vi "command change motor.vi"(8 "error in (no error)":errorcluster, 10 "the_command_change_motor":cluster{"Motor":u32}, 11 "id":i32) -> (0 "error out":errorcluster, 3 "function return":i32)   [LabVIEW 2012, in "libximc.lvlib"]
doc: "result_t XIMC_API command_change_motor (device_t id, const command_change_motor_t* the_command_change_motor);"
uses:
  libximc.lvlib
  libximc.dll
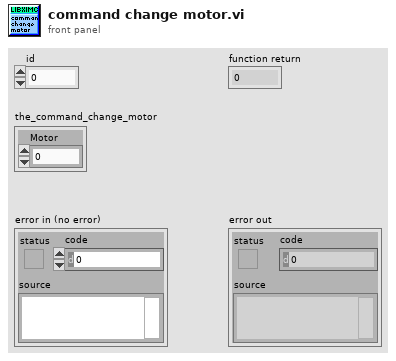
[diagram p1: front panel]
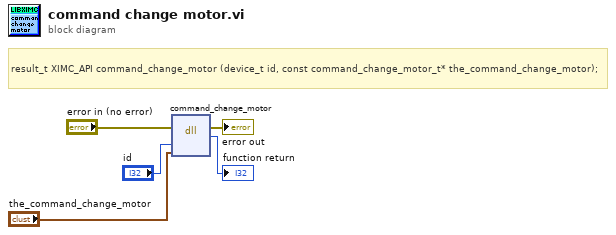
[diagram p0: block diagram]
diagram:
  # "result_t XIMC_API command_change_motor (device_t id, const command_change_motor_t* the_command_change_motor);"
  n1 = dll-call lib="E:/labview-2.12.1-Labview_12.0/ximcLVx32/libximc.*" fn="command_change_motor"(error in="error in (no error)", "id"="id", "the_command_change_motor"="the_command_change_motor") -> (error out=→"error out":errorcluster, →"function return":i32)  [unwired: 4 in, 1 out]
